vi "告警交互.vi"   [LabVIEW 2016, in "环境动力监测库.lvlib"]
types:
  T1 = cluster{"漏水监测输出":cluster{"漏水监测告警":bool, "告警内容":string}, "门禁监测输出":cluster{"门禁监测告警":bool, "告警内容":string}, "门禁监测输出2":cluster{"门禁监测告警":bool, "告警内容":string}, "温湿度监测输出":cluster{"温湿度监测告警":bool, "告警内容":string}, "烟雾监测输出":cluster{"烟雾监测告警":bool, "告警内容":string}, "空调监测输出":cluster{"空调监测告警":bool, "告警内容":string}, "自动重合闸输出":cluster{"自动重合闸告警":bool, "告警内容":string}, "红外入侵输出":cluster{"红外入侵告警":bool, "告警内容":string}, "振动输出":cluster{"振动告警":bool, "告警内容":string}, "UPS输出":cluster{"UPS告警":bool, "告警内容":string}, "蓄电池输出":cluster{"蓄电池告警":bool, "告警内容":string}, "蓄电池输出2":cluster{"蓄电池告警":bool, "告警内容":string}, "GPS输出":cluster{"定位告警":bool, "告警内容":string}, "北斗输出":cluster{"定位告警":bool, "告警内容":string}, "气象输出":cluster{"气象告警":bool, "告警内容":string}, "废液输出":cluster{"废液告警":bool, "告警内容":string}, "废液输出2":cluster{"废液告警":bool, "告警内容":string}}
  T2 = cluster{"温度告警":bool, "湿度告警":bool, "烟感告警":bool, "水浸告警":bool, "开门告警":bool}
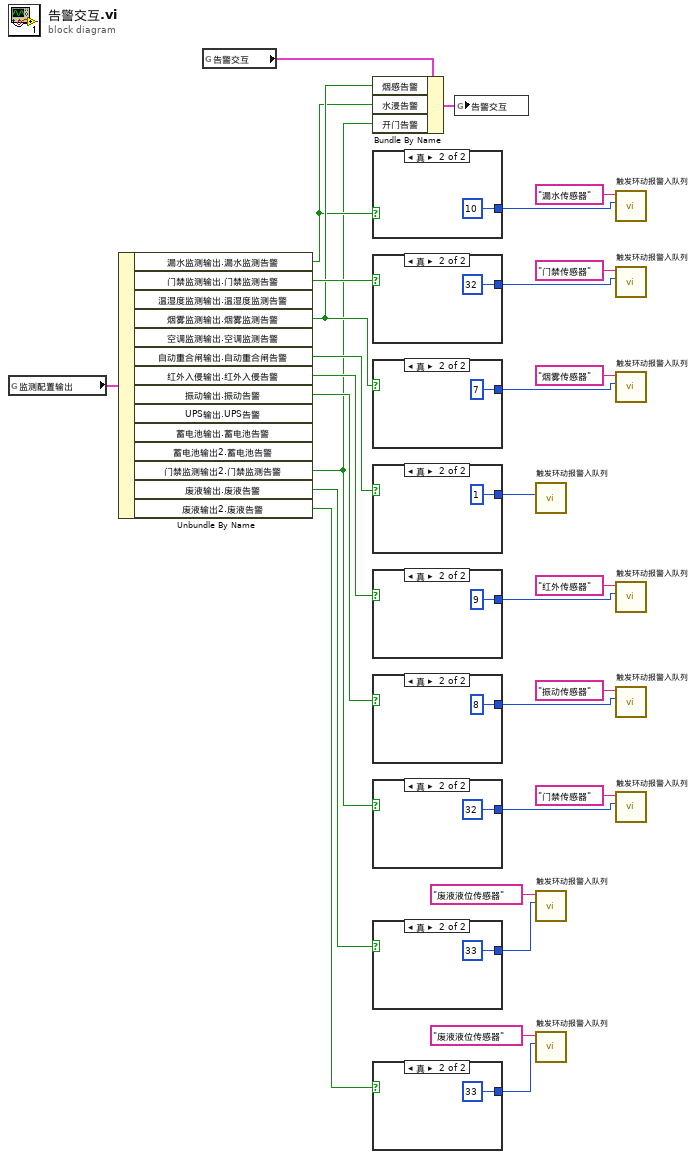
[diagram p0: block diagram]
diagram:
  n1 = global read "内部交互全局变量.vi" "监测配置输出"() -> (w29:T1)
  n2 = Unbundle By Name(w29) -> ("漏水监测输出.漏水监测告警"=w2:bool, "门禁监测输出.门禁监测告警"=w27:bool, "烟雾监测输出.烟雾监测告警"=w3:bool, "自动重合闸输出.自动重合闸告警"=w23:bool, "红外入侵输出.红外入侵告警"=w28:bool, "振动输出.振动告警"=w26:bool, "门禁监测输出2.门禁监测告警"=w1:bool, "废液输出.废液告警"=w25:bool, "废液输出2.废液告警"=w24:bool)  [unwired: 5 out]
  n3 = global read "外部交互全局变量.vi" "告警交互"() -> (w5:T2)
  n4 = Bundle By Name(cluster=w5, "烟感告警"=w3, "水浸告警"=w2, "开门告警"=w1) -> (w4:T2)
  n5 = case shown="真" w2 {
    tunnel: [_ 10 ("code")] -> w22
    frame False {
    }
    frame True {
    }
  }
  n6 = case shown="真" w27 {
    tunnel: [_ 32 ("code")] -> w20
    frame False {
    }
    frame True {
    }
  }
  n7 = case shown="真" w3 {
    tunnel: [_ 7 ("code")] -> w18
    frame False {
    }
    frame True {
    }
  }
  n8 = case shown="真" w23 {
    tunnel: [_ 1 ("code")] -> w16
    frame False {
    }
    frame True {
    }
  }
  n9 = case shown="真" w28 {
    tunnel: [_ 9 ("code")] -> w15
    frame False {
    }
    frame True {
    }
  }
  n10 = case shown="真" w26 {
    tunnel: [_ 8 ("code")] -> w13
    frame False {
    }
    frame True {
    }
  }
  n11 = case shown="真" w1 {
    tunnel: [_ 32 ("code")] -> w11
    frame False {
    }
    frame True {
    }
  }
  n12 = case shown="真" w25 {
    tunnel: [_ 33 ("code")] -> w9
    frame False {
    }
    frame True {
    }
  }
  n13 = case shown="真" w24 {
    tunnel: [_ 33 ("code")] -> w8
    frame False {
    }
    frame True {
    }
  }
  n14 = global write "外部交互全局变量.vi" "告警交互"(w4) -> ()
  n15 = call "触发环动报警入队列.vi"("code"=w16) -> ()  [unwired: 11 in]
  n16 = call "触发环动报警入队列.vi"("code"=w9, "元器件"="废液液位传感器") -> ()  [unwired: 10 in]
  n17 = call "触发环动报警入队列.vi"("code"=w8, "元器件"="废液液位传感器") -> ()  [unwired: 10 in]
  n18 = call "触发环动报警入队列.vi"("code"=w22, "元器件"="漏水传感器") -> ()  [unwired: 10 in]
  n19 = call "触发环动报警入队列.vi"("code"=w20, "元器件"="门禁传感器") -> ()  [unwired: 10 in]
  n20 = call "触发环动报警入队列.vi"("code"=w18, "元器件"="烟雾传感器") -> ()  [unwired: 10 in]
  n21 = call "触发环动报警入队列.vi"("code"=w15, "元器件"="红外传感器") -> ()  [unwired: 10 in]
  n22 = call "触发环动报警入队列.vi"("code"=w13, "元器件"="振动传感器") -> ()  [unwired: 10 in]
  n23 = call "触发环动报警入队列.vi"("code"=w11, "元器件"="门禁传感器") -> ()  [unwired: 10 in]
